vi "Extech_EX540_Reader.vi"(26 "read":bool=TRUE) -> (20 "read string":string="\n")   [LabVIEW 2013]
doc: "The Advanced Serial Read and Write example performs a Serial Port Read, a Serial Port Write, or a combination of these actions while setting some advanced serial features like buffer size, termination characters, and XON/XOFF flow control. The user selects the actions (read or write) on the front panel. If both are selected, the VI will write the data first, read the data and then close the VISA session that is opened to the port. \n\nThe parameters set for the serial port must match the parameters of the connected instrument or device. In this example, the bytes to read parameter specifies the number of bytes that the serial port reads. If there were more bytes at the port than the number specified in bytes to read, those bytes would not be read. Also, if you specify to read more bytes than the number of bytes actually read, you might receive a timeout error message.\n\nINSTRUCTIONS:\n1) Select the serial resource and configuration parameters (baud rate, data bits, parity, stop bits, flow control).\n2) Termination character can be enabled and set. Also, set the required input buffer size prior to running the example.\n3) Select the operations to be performed. \n4) Connect the serial port to your device. If no device is available, perform a loopback test by doing one of the following. Short pins 2 and 3 on a RS-232 cable or short pin 4 to pin 8 and pin 5 to pin 9 on a RS-485/422 cable. \n5) Run the VI to see the data read. (The \"read string\" will match the \"string to write\" if a loopback test was performed.)\n\nThis example exposes several advanced features that you may need for your application. Not all applications need all the features shown in this example. The input buffer size is likely an important setting that you want to control in your application. This example expands upon the flow control option for XON and XOFF, allowing the user to choose those control characters. The timeout parameter has been brought to the front panel so a user can specify the time period the VISA Read will wait for the number of bytes to read before timing out. Also, the user has several controls for the termination character, which is discussed later.\n\nNote that you can press the write and read buttons and change the bytes to read parameters on the fly, while the example is running. However, you must stop the example to change the other configuration parameters after the example has started running, and then run again.\n\nSet the I/O buffer size slightly higher the amount of data you expect to receive. This is very important for applications that don't use flow control, as you may lose characters if the receive buffer overflows.\n\nSetting the timeout period ensures that the operation returns with a timeout error if the operation cannot be performed in the specified time period. \n\nSome devices require a termination character in order to identify the end of command strings. Some devices send a termination character to signify the end of data to be read. \n\nThis example shows how you can end the Read operation once a termination character is detected in the buffer and/or append a termination character at the end of the Write data. To enable the Read to end on a termination character, use the VISA Configure Serial Port or use the VISA Properties Serial End Mode for Reads, Termination Character Enable, and Termination Character. To end the Write with a termination character, use the VISA Properties Serial End Mode for Writes, the Send End Enable, and Termination Character. In this example, the same termination character is used for both the Read and the Write. You can specify two different characters for your application, if desired.\n\nYour application may require specific characters for the XON/XOFF Flow Control. You can specify these characters with the VISA Properties Flow Control XOFF Character and Flow Control XON Character. Note that if the standard XON and XOFF characters are used, then decimal 17 and 19 are unavailable for data values. Remember that using flow control and setting an adequate buffer size allow you to prevent buffer overflows."
uses:
  <vilib>/Instr/_visa.llb/VISA Configure Serial Port (Instr).vi
  <vilib>/Utility/file.llb/Write To Spreadsheet File (string).vi
panel:
  out "AC + DC Mode":dbl
  out "Display Sign":dbl
  out "HOLD, REL, SIGN, PEAK":dbl
  out "Switch":dbl
  out "Mode":dbl
  out "Display Value":dbl format="%.3f"
  in  "stop":bool
  # "Extech EX540 Wireless Reader"
  # "Program Settings"
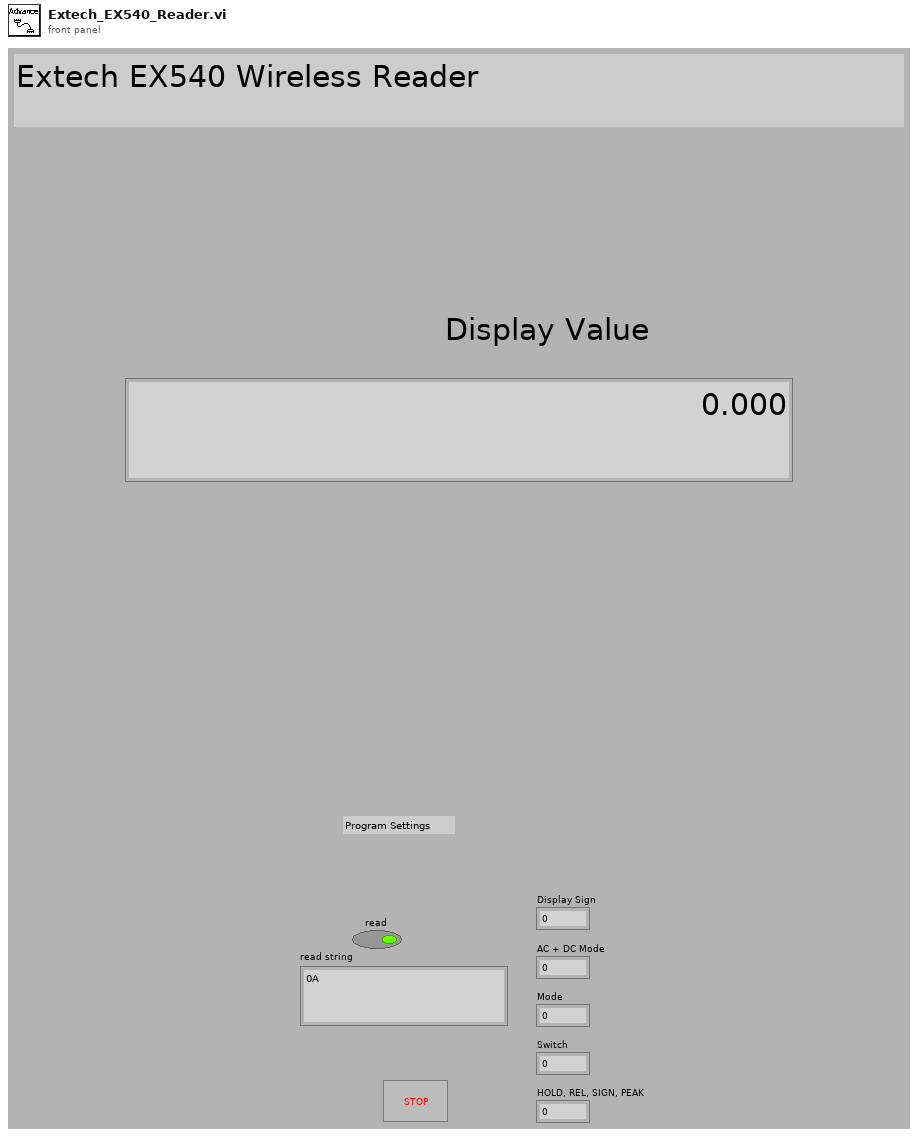
[diagram p1: front panel]
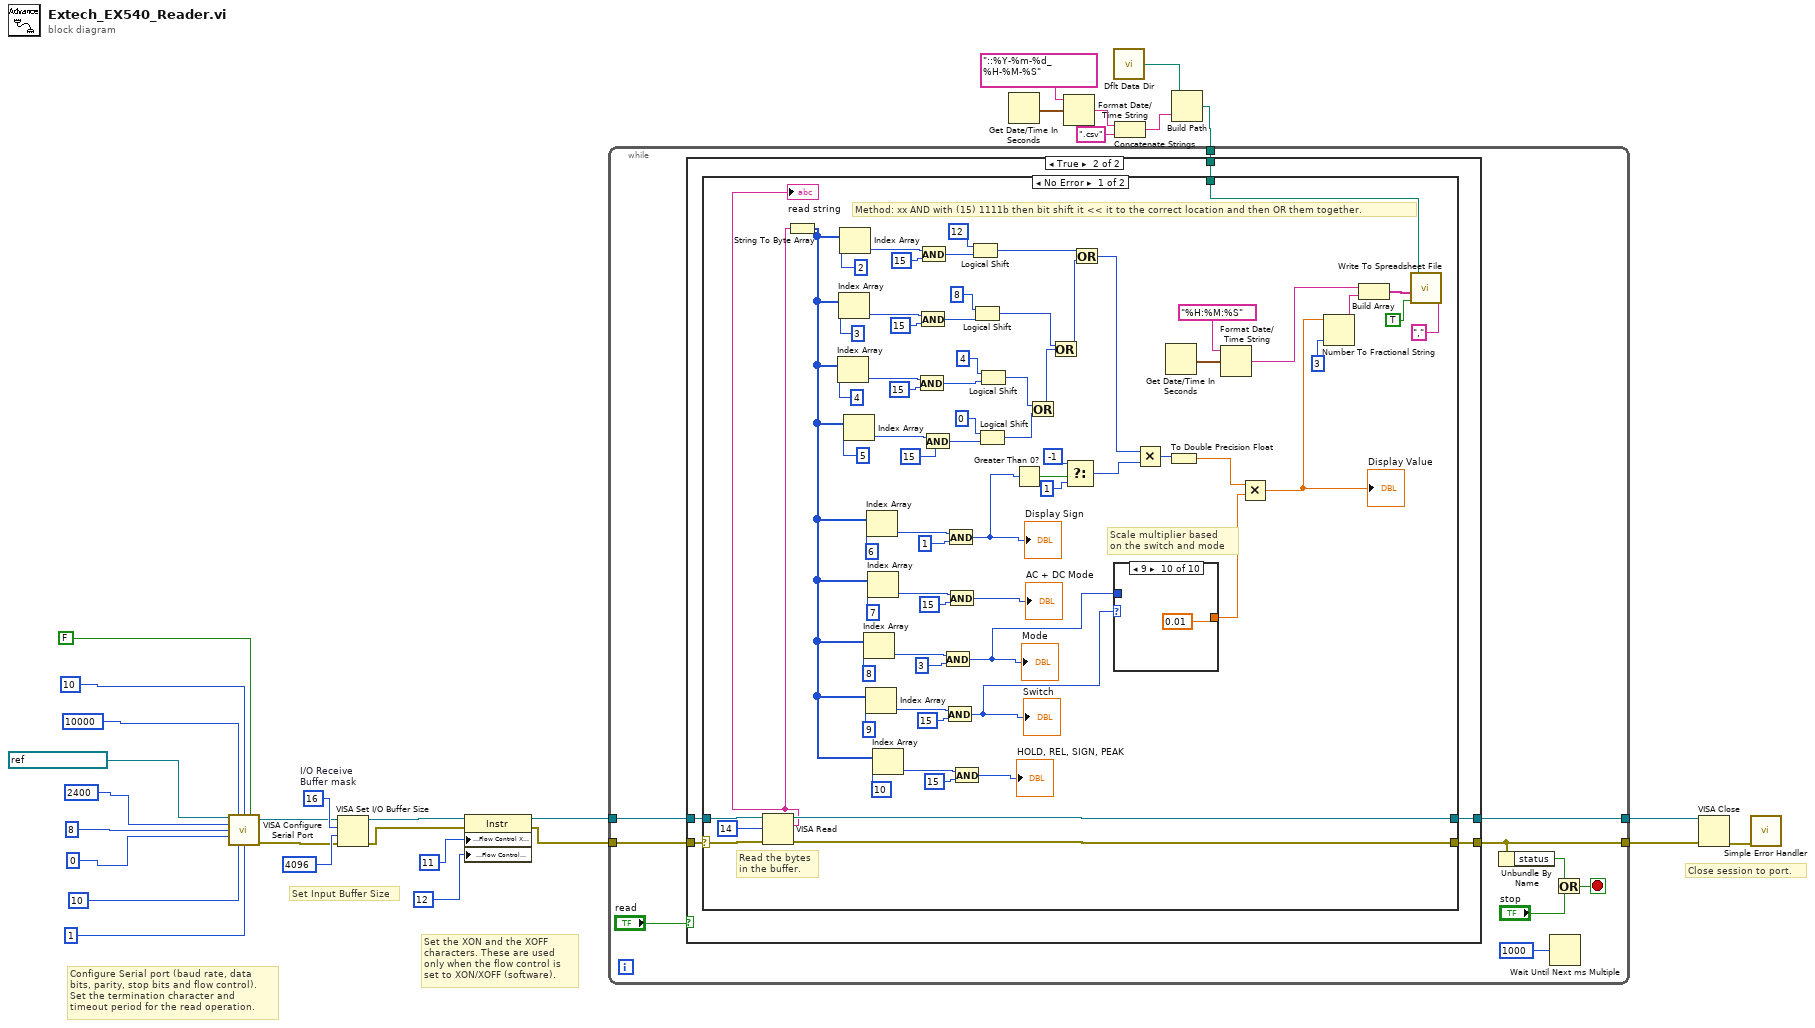
[diagram p0: block diagram]
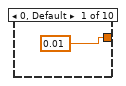
[diagram p3: hidden frame]
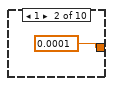
[diagram p4: hidden frame]
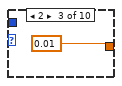
[diagram p5: hidden frame]
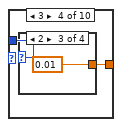
[diagram p6: hidden frame]
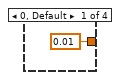
[diagram p7: hidden frame]
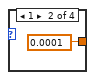
[diagram p8: hidden frame]
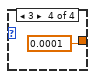
[diagram p9: hidden frame]
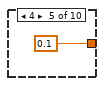
[diagram p10: hidden frame]
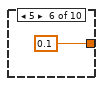
[diagram p11: hidden frame]
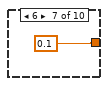
[diagram p12: hidden frame]
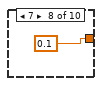
[diagram p13: hidden frame]
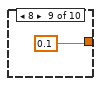
[diagram p14: hidden frame]
diagram:
  w27 = u16 16  # I/O Receive Buffer mask
  # "Set the XON and the XOFF\ncharacters. These are used\nonly when the flow control is\nset to XON/XOFF (software)."
  # "Configure Serial port (baud rate, data\nbits, parity, stop bits and flow control).\nSet the termination character and\ntimeout period for the read operation."
  # "Set Input Buffer Size"
  # "Close session to port."
  n1 = call-poly "VISA Configure Serial Port"("VISA resource name"=refnum<visa-resource-name> "ASRL1::INSTR", "timeout (10sec)"=u32 10000, "termination char\n(0xA = '\\n' = LF)"=10, "Enable Termination\nChar (T)"=FALSE, "baud rate (9600)"=2400, "data bits (8)"=8, "parity (0:none)"=0, "stop bits (10: 1 bit)"=u16 10, "flow control (0:none)"=1) -> ("VISA resource name out"=w12:refnum<visa-resource-name>, "error out"=w11:errorcluster)  [unwired: 5 in]
  n2 = VISA Set I/O Buffer Size(VISA resource name=w12, mask (16)=w27, size (4096)=4096, error in (no error)=w11) -> (VISA resource name out=w26:refnum<visa-resource-name>, error out=w25:errorcluster)
  n3 = property class="Instr"(reference=w26, error in=w25, "Serial Settings:Flow Control XON Character"=u8 11, "Serial Settings:Flow Control XOFF Character"=u8 12) -> (reference out=w23:refnum<visa-resource-name>, error out=w24:errorcluster)
  n4 = Get Date/Time In Seconds() -> (seconds since 1Jan1904=w7:timestamp)
  n5 = Format Date/Time String(time format string (%c)="::%Y-%m-%d_%H-%M-%S", seconds (now)=w7) -> (date/time string=w3:string)  [unwired: 1 in]
  n6 = call <vilib>:"Dflt Data Dir.vi"() -> ("App:Default Data Directory"=w4:path)
  n7 = Concatenate Strings(w3, ".csv" ("string")) -> (w1:string)
  n8 = Build Path(base path=w4, name or relative path=w1) -> (appended path=w5:path)
  n9 = while {
    tunnel: w24 -> [w32]
    tunnel: w23 -> [w33]
    tunnel: [w37] -> w22
    tunnel: [w36] -> w21
    tunnel: w5 -> [w30]
    stop <- w35 stop-if-true
    n10 = case shown="True" "read" {
      tunnel: w32 -> [w40 w44]
      tunnel: w33 -> [w41 w43]
      tunnel: [w40 w46] -> w36
      tunnel: [w41 w45] -> w37
      tunnel: w30 -> [_ w42]
      frame False {
      }
      frame True {
        n11 = case "Read bytes from port." shown="No Error" w44 {
          selector: w44 -> [w116 w133]
          tunnel: [w114 w133] -> w46
          tunnel: [w115 w134] -> w45
          tunnel: w43 -> [w117 w134]
          tunnel: w42 -> [w47 _]
          frame No Error {
            # "Method: xx AND with (15) 1111b then bit shift it << it to the correct location and then OR them together."
            # "Scale multiplier based\non the switch and mode"
            # "Read the bytes\nin the buffer."
            n12 = VISA Read(VISA resource name=w117, byte count=14, error in (no error)=w116) -> (VISA resource name out=w115:refnum<visa-resource-name>, read buffer=w62:string, error out=w114:errorcluster)  [unwired: 1 out]
            "read string" <- w62
            n13 = String To Byte Array(string=w62) -> (unsigned byte array=w112:u8[])
            n14 = Index Array(array=w112, index=4) -> (element=w73:u8)
            n15 = Index Array(array=w112, index=3) -> (element=w68:u8)
            n16 = Index Array(array=w112, index=2) -> (element=w65:u8)
            n17 = Index Array(array=w112, index=5) -> (element=w76:u8)
            n18 = Index Array(array=w112, index=8) -> (element=w91:u8)
            n19 = Index Array(array=w112, index=9) -> (element=w94:u8)
            n20 = Index Array(array=w112, index=6) -> (element=w101:u8)
            n21 = Index Array(array=w112, index=7) -> (element=w104:u8)
            n22 = Index Array(array=w112, index=10) -> (element=w97:u8)
            n23 = And(x=w73, y=15) -> (x .and. y?=w80:i32)
            n24 = And(x=w68, y=15) -> (x .and. y?=w77:i32)
            n25 = And(x=w65, y=15) -> (x .and. y?=w69:i32)
            n26 = And(x=w76, y=15) -> (x .and. y?=w82:i32)
            n27 = And(x=w91, y=3) -> (x .and. y?=w57:i32)
            "Mode" <- w57
            n28 = And(x=w94, y=15) -> (x .and. y?=w61:i32)
            "Switch" <- w61
            n29 = And(x=w101, y=1) -> (x .and. y?=w106:i32)
            "Display Sign" <- w106
            n30 = And(x=w104, y=15) -> (x .and. y?=→"AC + DC Mode":i32)
            n31 = And(x=w97, y=15) -> (x .and. y?=→"HOLD, REL, SIGN, PEAK":i32)
            n32 = Logical Shift(y=12, x=w69) -> (x << y=w88:i32)
            n33 = Logical Shift(y=8, x=w77) -> (x << y=w86:i32)
            n34 = Logical Shift(y=0, x=w82) -> (x << y=w83:i32)
            n35 = Logical Shift(y=4, x=w80) -> (x << y=w84:i32)
            n36 = Greater Than 0?(x=w106) -> (x > 0?=w107:bool)
            n37 = Or(x=w84, y=w83) -> (x .or. y?=w85:i32)
            n38 = Or(x=w86, y=w85) -> (x .or. y?=w87:i32)
            n39 = Select(t=-1, s=w107, f=1) -> (s? t:f=w110:i32)
            n40 = Or(x=w88, y=w87) -> (x .or. y?=w111:i32)
            n41 = case shown="9" w61 {
              tunnel: [0.01 0.0001 0.01 w121 0.1 0.1 0.1 0.1 0.1 0.01] -> w59
              tunnel: w57 -> [_ _ _ w122 _ _ _ _ _ _]
              frame 0, Default {
              }
              frame 1 {
              }
              frame 2 {
              }
              frame 3 {
                n42 = case shown="2" w122 {
                  tunnel: [0.01 0.0001 0.01 0.0001] -> w121
                  frame 0, Default {
                  }
                  frame 1 {
                  }
                  frame 2 {
                  }
                  frame 3 {
                  }
                }
              }
              frame 4 {
              }
              frame 5 {
              }
              frame 6 {
              }
              frame 7 {
              }
              frame 8 {
              }
              frame 9 {
              }
            }
            n43 = Multiply(x=w111, y=w110) -> (x*y=w60:i32)
            n44 = Get Date/Time In Seconds() -> (seconds since 1Jan1904=w54:timestamp)
            n45 = To Double Precision Float(number=w60) -> (double precision float=w58:dbl)
            n46 = Format Date/Time String(time format string (%c)="%H:%M:%S", seconds (now)=w54) -> (date/time string=w53:string)  [unwired: 1 in]
            n47 = Multiply(x=w58, y=w59) -> (x*y=w49:dbl)
            "Display Value" <- w49
            n48 = Number To Fractional String(number=w49, precision (6)=i16 3) -> (F-format string=w50:string)  [unwired: 2 in]
            n49 = Build Array(w53, w50) -> (w55:string[])
            n50 = call-poly <vilib>:"Write To Spreadsheet File.vi"("delimiter (\\t)"="," ("delimiter (\\t)"), "append to file? (new file:F)"=TRUE, "1D data"=w55, "file path (dialog if empty)"=w47) -> ()  [unwired: 4 in, 1 out]
          }
          frame Error {
            # "Error occurred \nreading Bytes at \nSerial Port"
          }
        }
      }
    }
    n51 = Unbundle By Name(w36) -> ("status"=w38:bool)
    n52 = Wait Until Next ms Multiple(millisecond multiple=u32 1000) -> ()  [unwired: 1 out]
    n53 = Or(x=w38, y="stop") -> (x .or. y?=w35:bool)
  }
  n54 = VISA Close(VISA resource name=w22, error in (no error)=w21) -> (error out=w28:errorcluster)
  n55 = call <vilib>:"Simple Error Handler.vi"("error in (no error)"=w28) -> ()  [unwired: 4 in, 5 out]
